vi "gu_move.vi"(8 "error in":errorcluster, 10 "Destination Path":T1, 11 "Source Path":T1) -> (0 "error out":errorcluster)   [LabVIEW 2020, in "G-Unicode.lvlib"]
uses:
  G-Unicode.lvlib
  Types/Encoded UTF-8 String.ctl
  lib/g_unicode_32.dll
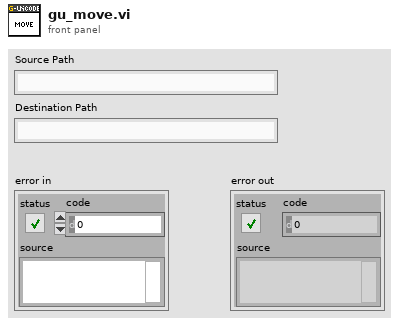
[diagram p1: front panel]
types:
  T1 = typedef "G-Unicode.lvlib/Encoded UTF-8 String.ctl" = string
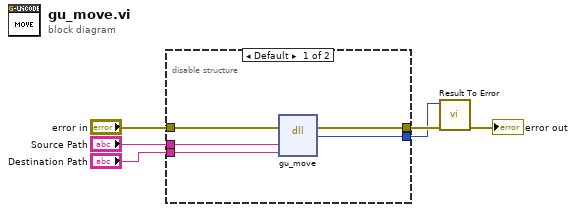
[diagram p0: block diagram]
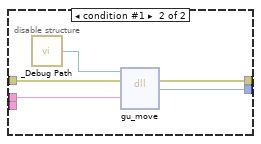
[diagram p2: hidden frame]
diagram:
  n1 = disable-structure shown="Default" {
    disable-tunnel: [w11 w16] -> w6
    disable-tunnel: [w10 w15] -> w1
    disable-tunnel: "Source Path" -> [w9 w14]
    disable-tunnel: "error in" -> [w8 w13]
    disable-tunnel: "Destination Path" -> [w7 _]
    frame condition #0 (active) {
      n2 = dll-call lib="C:/github/dataflowg/g-unicode/src/LabVIEW/G-Unicode/lib/g_unicode_*.*" fn="gu_move"(error in=w8, "source_path"=w9, "dest_path"=w7) -> (error out=w11:errorcluster, "result"=w10:i32)  [unwired: 4 in, 1 out]
    }
    frame condition #1 {
      n3 = call "_Debug Path.vi"() -> ("Debug Path"=w12:path)
      n4 = dll-call lib="?" fn="gu_move"(path in=w12, error in=w13, "source_path"=w14) -> (error out=w16:errorcluster, "result"=w15:i32)  [unwired: 4 in, 1 out]
    }
  }
  n5 = call "Result To Error.vi"("error in (no error)"=w6, "Result Code"=w1) -> ("error out"=→"error out":errorcluster)  [unwired: 9 in]
